vi "StartPath.vi"(11 "PathFileRef In":T1) -> (3 "PathFileRef Out":T1)   [LabVIEW 2014]
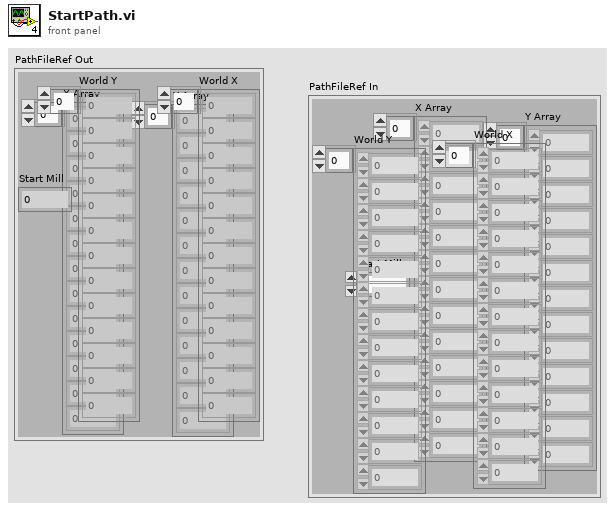
[diagram p1: front panel]
types:
  T1 = cluster{"X Array":dbl[], "Y Array":dbl[], "Start Mill":i32, "World X":dbl[], "World Y":dbl[]}
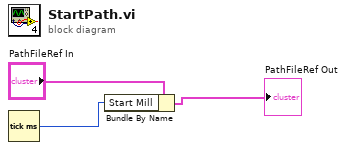
[diagram p0: block diagram]
diagram:
  n1 = Tick Count (ms)() -> (millisecond timer value=w1:u32)
  n2 = Bundle By Name(cluster="PathFileRef In", "Start Mill"=w1) -> (→"PathFileRef Out":T1)
